vi "Module Init.vi"(8 "error in (no error)":errorcluster, 11 "Historian Logger in":refnum<class "Historian Logger.lvclass">) -> (0 "error out":errorcluster, 3 "Historian Logger out":refnum<class "Historian Logger.lvclass">)   [LabVIEW 2020, in "VolatusHistorian.lvlib" / "Historian Logger.lvclass"]
uses:
  Historian Logger.lvclass
  Historian Logger.lvclass/Historian Logger.ctl
  Volatus/Module/Module.lvclass
  C:/dev/lv20CE/relink/lv-volatus/Volatus/Module/Module.lvclass
  C:/dev/lv20CE/relink/lv-volatus/VolatusHistorian/Historian Logger/Historian Logger.lvclass
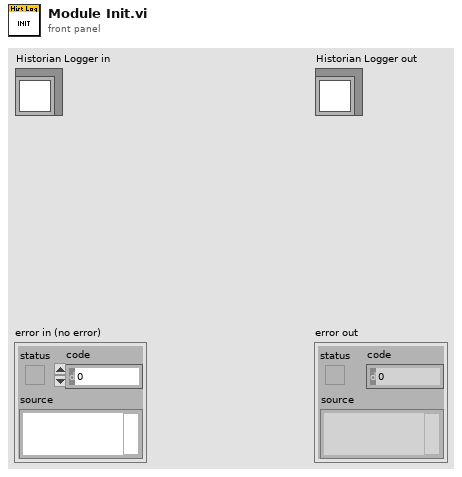
[diagram p1: front panel]
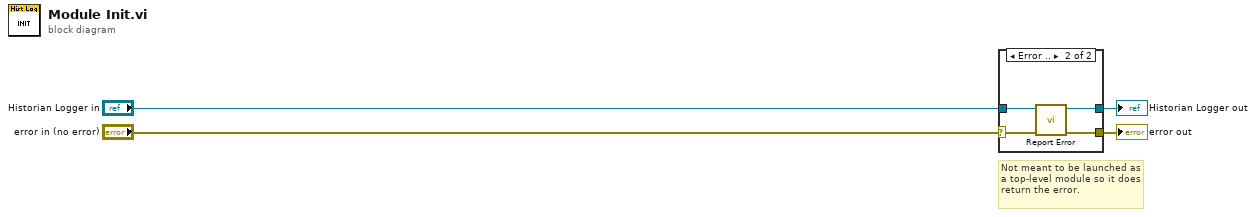
[diagram p0: block diagram]
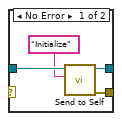
[diagram p2: hidden frame]
diagram:
  # "Not meant to be launched as a top-level module so it does return the error."
  n1 = case shown="Error .." "error in (no error)" {
    selector: "error in (no error)" -> [_ w11]
    tunnel: [w8 w9] -> w3
    tunnel: "Historian Logger in" -> [w7 w12]
    tunnel: [w6 w10] -> w1
    frame No Error {
      n2 = call "Send to Self.vi"("Message ID"="Initialize", "Module in"=w7) -> ("error out"=w8:errorcluster, "Module out"=w6:refnum<class "Historian Logger.lvclass">)  [unwired: 8 in]
    }
    frame Error {
      n3 = call "Report Error.vi"("error in (no error)"=w11, "Module in"=w12) -> ("error out"=w9:errorcluster, "Module out"=w10:refnum<class "Historian Logger.lvclass">)  [unwired: 8 in]
    }
  }
  "error out" <- w3
  "Historian Logger out" <- w1
